vi "Init Map to Outgoing Frame Configs.vi"(7 "error in (no error)":errorcluster, 10 "RT Configuration In":T1={"Name"="", "Priority"=100, "XNET Settings"={"Database"="", "Cluster"="", "Port"="", "Baud rate [Bd]"=0, "Termination"=0, "CAN I/O Mode"=0, "FD Baud rate [Bd]"=500000, "Priority"=100, "Use Legacy"=FALSE, "FD ISO Mode"=0}, "FPGA Session"=0, "Outgoing CAN Session"="", "Outgoing Frame Count"=0, "Outgoing Frames"=[], "Incoming CAN Session"="", "Incoming Frame Count"=0, "Incoming Frames"=[], "Incoming Values"={"Signal Values"=[], "Signal Invalid Values"=[], "ProtCtr Sig Values"=[], "Timestamps"=[], "Time Differences"=[], "IDs"=[]}} {"Incoming Frames"."Protection Configurations"."CRC Channels"."Data Type" items=["Signed", "Unsigned", "IEEE Float"]; "XNET Settings"."FD ISO Mode" items=["ISO", "Non ISO", "ISO Legacy"]; "XNET Settings"."CAN I/O Mode" items=["CAN 2.0", "CAN FD", "CAN FD+BRS"]; "XNET Settings"."Termination" items=["Off", "On"]; "Outgoing Frames"."Protection Configurations"."CRC Channels"."Data Type" items=["Signed", "Unsigned", "IEEE Float"]}) -> (0 "error out":errorcluster, 2 "Map":map{i32, u8[]}(c390), 3 "RT Configuration Out":T1={"Name"="", "Priority"=100, "XNET Settings"={"Database"="", "Cluster"="", "Port"="", "Baud rate [Bd]"=0, "Termination"=0, "CAN I/O Mode"=0, "FD Baud rate [Bd]"=500000, "Priority"=100, "Use Legacy"=FALSE, "FD ISO Mode"=0}, "FPGA Session"=0, "Outgoing CAN Session"="", "Outgoing Frame Count"=0, "Outgoing Frames"=[], "Incoming CAN Session"="", "Incoming Frame Count"=0, "Incoming Frames"=[], "Incoming Values"={"Signal Values"=[], "Signal Invalid Values"=[], "ProtCtr Sig Values"=[], "Timestamps"=[], "Time Differences"=[], "IDs"=[]}} {"Incoming Frames"."Protection Configurations"."CRC Channels"."Data Type" items=["Signed", "Unsigned", "IEEE Float"]; "XNET Settings"."FD ISO Mode" items=["ISO", "Non ISO", "ISO Legacy"]; "XNET Settings"."CAN I/O Mode" items=["CAN 2.0", "CAN FD", "CAN FD+BRS"]; "XNET Settings"."Termination" items=["Off", "On"]; "Outgoing Frames"."Protection Configurations"."CRC Channels"."Data Type" items=["Signed", "Unsigned", "IEEE Float"]})   [LabVIEW 2023, in "LP_CRC.lvlib"]
uses:
  LP_CRC.lvlib
  Addon/Addon Engine/Types/RT Async Engine Settings.ctl
  Addon/Addon Shared/Types/XNET Settings.ctl
  Engine/Types/RT Frame Settings.ctl
  Shared/Types/Exported Frame Type.ctl
  Engine/Types/RT Protection Configuration.ctl
  Shared/Types/Protection Type.ctl
  Shared/Types/XNET Signal Configuration.ctl
  Shared/Types/Exported Counter Settings.ctl
  Shared/Types/Exported Event Trigger Type.ctl
  Engine/Types/RT Frame Incoming Values.ctl
  Shared/Protection and Counter Support Shared.lvlib
  Engine/Protection and Counter Support Engine.lvlib
  Addon/Addon Shared/Protection and Counter Addon Shared.lvlib
  Addon/Addon Engine/Protection and Counter Addon Engine.lvlib
panel:
  in  "key names":string[](array[string])=["22E", "2AA", "2AB", "FC", "231", "234", "E1", "22F", "232", "1A1", "13A", "CA", "DB", "316", "324", "BD", "13B", "233", "2A3", "228", "22A", "18D", "0B1", "0B2", "137", "138", "182", "183", "184", "185", "186", "18C", "227", "3CE", "FA", "FD", "25A", "B1", "B2", "B6", "B7", "2C0", "381", "181", "235", "3BA", "2AD", "2AC", "3C3", "3C2", "3C5", "305", "30B", "30C", "50", "201-214", "215-21E", "200", "21F", "52", "30", "120-12F", "14D", "190-19F", "1C0-1CF", "14C", "170-17F"]
  in  "key values":string[](array[string])=["0x8D, 0xBB, 0x4E, 0x7B, 0xE9, 0xCE, 0x31, 0x61, 0x7C, 0xB0, 0xA5, 0x3, 0x81, 0xC5, 0x84, 0x4B", "0x62, 0xB4, 0x14, 0x71, 0x7C, 0x99, 0xA1, 0xD, 0x49, 0x8B, 0x95, 0xB, 0x43, 0x94, 0x4, 0xC2", "0xD2, 0x6A, 0x4A, 0xB0, 0x9F, 0xCD, 0x65, 0x4E, 0xB4, 0xE0, 0x4C, 0x16, 0x37, 0x1C, 0xE8, 0x22", "0x8B, 0x8, 0xF1, 0x2B, 0xD3, 0x87, 0x93, 0xEE, 0x55, 0xAB, 0xC3, 0xDA, 0x91, 0x77, 0x9E, 0x3", "0x3F, 0xF1, 0xC6, 0xD5, 0xB, 0x99, 0x6F, 0xEB, 0x41, 0xF5, 0x56, 0xA2, 0xAD, 0x7, 0xCC, 0x4E", "0x45, 0xEF, 0xBA, 0xF9, 0x6B, 0xAA, 0xCC, 0x37, 0x8C, 0x74, 0x6, 0x20, 0x55, 0x5C, 0xD7, 0x57", "0x25, 0xF8, 0x32, 0xEC, 0x4F, 0x53, 0xB4, 0xC4, 0xF9, 0x30, 0x4, 0x58, 0x3E, 0x86, 0x63, 0xF6", "0x91, 0xCA, 0xEC, 0x22, 0xB2, 0xC4, 0x69, 0xCF, 0x58, 0x1B, 0x99, 0xF6, 0x9A, 0x46, 0xB9, 0xC9", "0x10, 0xBD, 0x87, 0x75, 0xF7, 0x6D, 0x42, 0x55, 0xC5, 0xC0, 0x25, 0x4C, 0xDA, 0x70, 0x40, 0x1D", "0x19, 0x8F, 0x31, 0x8D, 0x96, 0x1D, 0x67, 0x9, 0xFB, 0x66, 0xB4, 0x39, 0x10, 0xD4, 0xF6, 0xF2", "0x55, 0xAA, 0x46, 0x3C, 0x26, 0xED, 0x81, 0xCA, 0x38, 0x3E, 0xDD, 0x11, 0xA7, 0x7C, 0x1E, 0x2A", "0x98, 0x34, 0xBE, 0x86, 0x6D, 0xE, 0x89, 0x1F, 0x2B, 0x69, 0x74, 0x4D, 0xB4, 0x68, 0x44, 0x12", "0xF8, 0xBE, 0x8, 0xE, 0xF2, 0x2B, 0xC1, 0x4D, 0x87, 0x44, 0x6B, 0xEE, 0x14, 0x60, 0xAB, 0x19", "0x66, 0x7, 0x97, 0xF4, 0x23, 0x51, 0xA8, 0x2, 0x76, 0xC8, 0x8, 0x48, 0xBB, 0x52, 0x53, 0xA7", "0x2B, 0xEE, 0xDA, 0x3, 0x30, 0x32, 0x9F, 0x31, 0x3C, 0xAE, 0x5F, 0xBB, 0xD5, 0xE0, 0x33, 0x1D", "0x4C, 0xA3, 0xA1, 0x2C, 0xA4, 0x21, 0x6, 0x98, 0x97, 0x49, 0x58, 0x13, 0x28, 0x8F, 0x68, 0xDB", "0xA5, 0x5A, 0x88, 0x77, 0x50, 0x5F, 0xEF, 0xEA, 0x4D, 0x3F, 0xA3, 0xCD, 0x8E, 0xF9, 0xE1, 0x2E", "0xA5, 0xE9, 0x85, 0x4, 0xFB, 0x6C, 0xDF, 0xF1, 0xDE, 0x90, 0xA8, 0xCB, 0xDD, 0x3B, 0x80, 0x87", "0x14, 0x99, 0x49, 0xB, 0x4, 0xD5, 0x74, 0xC6, 0x17, 0xF1, 0xE1, 0x3F, 0x50, 0x9B, 0xCB, 0x10", "0xC5, 0x9E, 0x5D, 0xA1, 0xAC, 0x96, 0x1B, 0x21, 0x82, 0xEE, 0xF9, 0x97, 0xB1, 0xCB, 0xB6, 0x13", "0xD5, 0xEB, 0xA2, 0x4E, 0x35, 0xAE, 0x51, 0xCE, 0x2D, 0x79, 0x9F, 0x7C, 0x34, 0x52, 0x9, 0x3", "0x61, 0x4B, 0x17, 0xE4, 0x78, 0xB, 0xA1, 0xB4, 0xBC, 0xD8, 0xEA, 0xF5, 0xD9, 0x21, 0xCA, 0x86", "0x49, 0x56, 0xE, 0x67, 0x81, 0x1E, 0x76, 0x9F, 0xBF, 0xC1, 0xE5, 0x6C, 0x96, 0x83, 0x7F, 0xC2", "0x9C, 0xD6, 0x1C, 0xBA, 0xB8, 0x8, 0xAB, 0xAA, 0x49, 0xDF, 0x1B, 0x8C, 0x6D, 0x6E, 0xEA, 0x20", "0x57, 0x39, 0x72, 0xD, 0x51, 0xB1, 0x25, 0x28, 0x5A, 0x52, 0x85, 0xB8, 0x38, 0xF8, 0x2B, 0x6B", "0xC1, 0x5, 0xD2, 0xD9, 0xAE, 0x93, 0xB1, 0x90, 0x42, 0x7C, 0x60, 0x33, 0x46, 0xB8, 0x6A, 0xE1", "0xE8, 0x40, 0x60, 0xDE, 0xC2, 0xAC, 0xE3, 0xA4, 0x3D, 0x88, 0xD1, 0xEE, 0x51, 0x16, 0xAD, 0x49", "0xF7, 0xC0, 0x40, 0xA6, 0xA5, 0xDE, 0x62, 0x1C, 0xAC, 0x5A, 0x4F, 0xA4, 0xE5, 0x18, 0x88, 0x8", "0xD9, 0x90, 0x33, 0xE1, 0x3A, 0x1A, 0xDF, 0xC6, 0xB5, 0xDC, 0xEE, 0x4, 0xFA, 0xD7, 0xD4, 0x99", "0x5D, 0x96, 0x82, 0x97, 0xB6, 0x8B, 0x24, 0x2, 0xEB, 0x69, 0x20, 0xBB, 0x77, 0x54, 0x86, 0xE6", "0xD3, 0xE0, 0x75, 0x85, 0x83, 0x55, 0x33, 0xE3, 0x4C, 0x9C, 0x91, 0x1D, 0x23, 0x1A, 0xA6, 0x16", "0xF, 0xD1, 0x6B, 0x63, 0x9E, 0x74, 0x22, 0x94, 0xD7, 0xA1, 0xE7, 0x6F, 0x9C, 0xCF, 0x96, 0xDD", "0x66, 0xF4, 0xA8, 0xC8, 0xBB, 0xA7, 0xAF, 0x2B, 0xD9, 0x7B, 0xC0, 0x50, 0x56, 0xF, 0xCE, 0xED", "0x6C, 0x14, 0x3C, 0xAD, 0x93, 0x59, 0x1C, 0x4D, 0xD8, 0x33, 0x5D, 0x89, 0x7B, 0x8, 0x70, 0x34", "0x96, 0x97, 0x8B, 0x2, 0x69, 0xBB, 0x54, 0xE6, 0x4E, 0x46, 0x8D, 0x7B, 0xEA, 0x87, 0xE9, 0xB3", "0x53, 0x58, 0x37, 0xDA, 0x94, 0x57, 0x79, 0x27, 0x8D, 0xDD, 0xD0, 0x39, 0x16, 0x84, 0x7, 0xAF", "0x64, 0x5D, 0x7D, 0x96, 0x3D, 0x82, 0xB9, 0x97, 0xD5, 0xB6, 0xAA, 0x8B, 0x5A, 0x24, 0xB4, 0x2", "0x49, 0x56, 0xE, 0x67, 0x81, 0x1E, 0x76, 0x9F, 0xBF, 0xC1, 0xE5, 0x6C, 0x96, 0x83, 0x7F, 0xC2", "0x9C, 0xD6, 0x1C, 0xBA, 0xB8, 0x8, 0xAB, 0xAA, 0x49, 0xDF, 0x1B, 0x8C, 0x6D, 0x6E, 0xEA, 0x20", "0x71, 0xD, 0xB, 0xC2, 0x8, 0xC6, 0x63, 0x4B, 0x3F, 0x2B, 0x6, 0x10, 0xF0, 0xD2, 0x87, 0xD", "0xEB, 0x4E, 0xAE, 0xCE, 0x79, 0x7C, 0x52, 0x3, 0x6A, 0x84, 0xC2, 0x3A, 0xA, 0x64, 0x2F, 0x17", "0xA3, 0x4F, 0xD2, 0xB1, 0x60, 0x6A, 0x36, 0xF5, 0x4A, 0xAF, 0xED, 0xB0, 0x57, 0xF6, 0x9F, 0xAD", "0xB2, 0x18, 0xB8, 0xA, 0xA4, 0xD0, 0xBA, 0x5A, 0xD4, 0x54, 0x1C, 0x95, 0xB1, 0xDE, 0xD6, 0xF", "0xC8, 0x83, 0x64, 0xF, 0xC7, 0xB7, 0x3F, 0x2D, 0x68, 0x57, 0x30x, 0x88, 0x1C, 0xF7, 0x5C, 0x1A", "0xA8, 0xA7, 0xD9, 0x50, 0xCE, 0x90, 0x28, 0x3F, 0x33, 0x3, 0xDE, 0xE1, 0x1E, 0x6B, 0x3A, 0xF1", "0xB3, 0x67, 0x98, 0xD4, 0x82, 0x34, 0x53, 0x72, 0xBE, 0xF0, 0xA1, 0x86, 0x4A, 0x64, 0x6D, 0xE1", "0x31, 0x1D, 0xFB, 0x39, 0xF6, 0x90, 0x34, 0xD3, 0x80, 0x97, 0x99, 0x2F, 0x5E, 0x86, 0x1C, 0xAB", "0xE4, 0xB4, 0xF5, 0x86, 0xC, 0x35, 0x13, 0xE9, 0x5C, 0xF3, 0x5B, 0x79, 0xE1, 0x43, 0xCF, 0xB0", "0x14, 0xAD, 0x59, 0x4D, 0x33, 0x89, 0x8, 0x34, 0xC, 0x1A, 0x96, 0x11, 0x61, 0x8C, 0xB5, 0xA", "0x5, 0xD9, 0x93, 0x90, 0x7C, 0x33, 0xB8, 0xE1, 0x70, 0x3A, 0xAC, 0x1A, 0xBF, 0xDF, 0x9A, 0xC6", "0x51, 0x52, 0x2B, 0x64, 0xB3, 0xED, 0x4F, 0x5D, 0x3F, 0x80, 0xD6, 0x7D, 0xF2, 0x30, 0x4B, 0x96", "0x6A, 0xB0, 0xCD, 0x4E, 0xE0, 0x16, 0x1C, 0x22, 0x71, 0x98, 0xD9, 0xDF, 0xFA, 0x76, 0xF8, 0x14", "0x5B, 0xA8, 0x5, 0xA7, 0x4E, 0xD9, 0xD, 0x50, 0x93, 0xCE, 0x40, 0x90, 0xE, 0x28, 0x7C, 0x3F", "0xD8, 0x8E, 0x56, 0x3A, 0x18, 0xCC, 0xC9, 0x53, 0x15, 0xA, 0x90, 0x8A, 0x3E, 0x7A, 0xD0, 0x64", "0xBC, 0xEB, 0xB1, 0x41, 0x29, 0xF5, 0x66, 0x56, 0xB0, 0xA2, 0xCA, 0xAD, 0x1, 0x7, 0xB3, 0xCC", "0x27, 0xDC, 0x8D, 0x50, 0xDD, 0x9, 0xD0, 0x6D, 0x39, 0x21, 0x16, 0xF2, 0x84, 0x95, 0x7, 0x69", "0x27, 0xDC, 0x8D, 0x50, 0xDD, 0x9, 0xD0, 0x6D, 0x39, 0x21, 0x16, 0xF2, 0x84, 0x95, 0x7, 0x69", "0xF1, 0x87, 0x55, 0xDA, 0x9E, 0xAA, 0xB5, 0x32, 0x46, 0x7F, 0x2C, 0x3C, 0x7A, 0x1B, 0x26, 0xBB", "0xD9, 0xC7, 0x9A, 0x57, 0xD7, 0x5C, 0x55, 0x20, 0x6, 0x74, 0x8C, 0x37, 0xCC, 0xAA, 0x6B, 0xF9", "0x38,0x4C, 0xA, 0xD9, 0x7D, 0x5A, 0x6C, 0xC7, 0x95, 0xC4, 0x51, 0x9A, 0x41, 0xCB, 0xC0, 0x57", "0x93, 0x77, 0xB5, 0x9F, 0xB6, 0x1B, 0x41, 0xE0, 0x81, 0x27, 0x78, 0xE8, 0x6B, 0x56, 0x8F, 0x98", "0x1F, 0xB6, 0x19, 0x27, 0x9C, 0x8F, 0xA2, 0xDC, 0x31, 0xCF, 0x4A, 0x8D, 0xC2, 0xB8, 0x96, 0x50", "0xE5, 0xBA, 0xC8, 0xDE, 0xA9, 0x83, 0xB, 0xC, 0x64, 0x79, 0x44, 0xF, 0xF6, 0xC6, 0xC7, 0x5", "0x68, 0x29, 0xAF, 0xA2, 0xEF, 0xB3, 0x5B, 0xB8, 0xE0, 0x59, 0x7E, 0x67, 0x63, 0x23, 0x43, 0xD0", "0x68, 0x29, 0xAF, 0xA2, 0xEF, 0xB3, 0x5B, 0xB8, 0xE0, 0x59, 0x7E, 0x67, 0x63, 0x23, 0x43, 0xD0", "0x6C, 0xCB, 0xC, 0x55, 0xEA, 0x5, 0x4B, 0xAA, 0x2D, 0x28, 0x9C, 0x46, 0xF4, 0x84, 0x1, 0x3C", "0x1F, 0xB6, 0x19, 0x27, 0x9C, 0x8F, 0xA2, 0xDC, 0x31, 0xCF, 0x4A, 0x8D, 0xC2, 0xB8, 0x96, 0x50"]
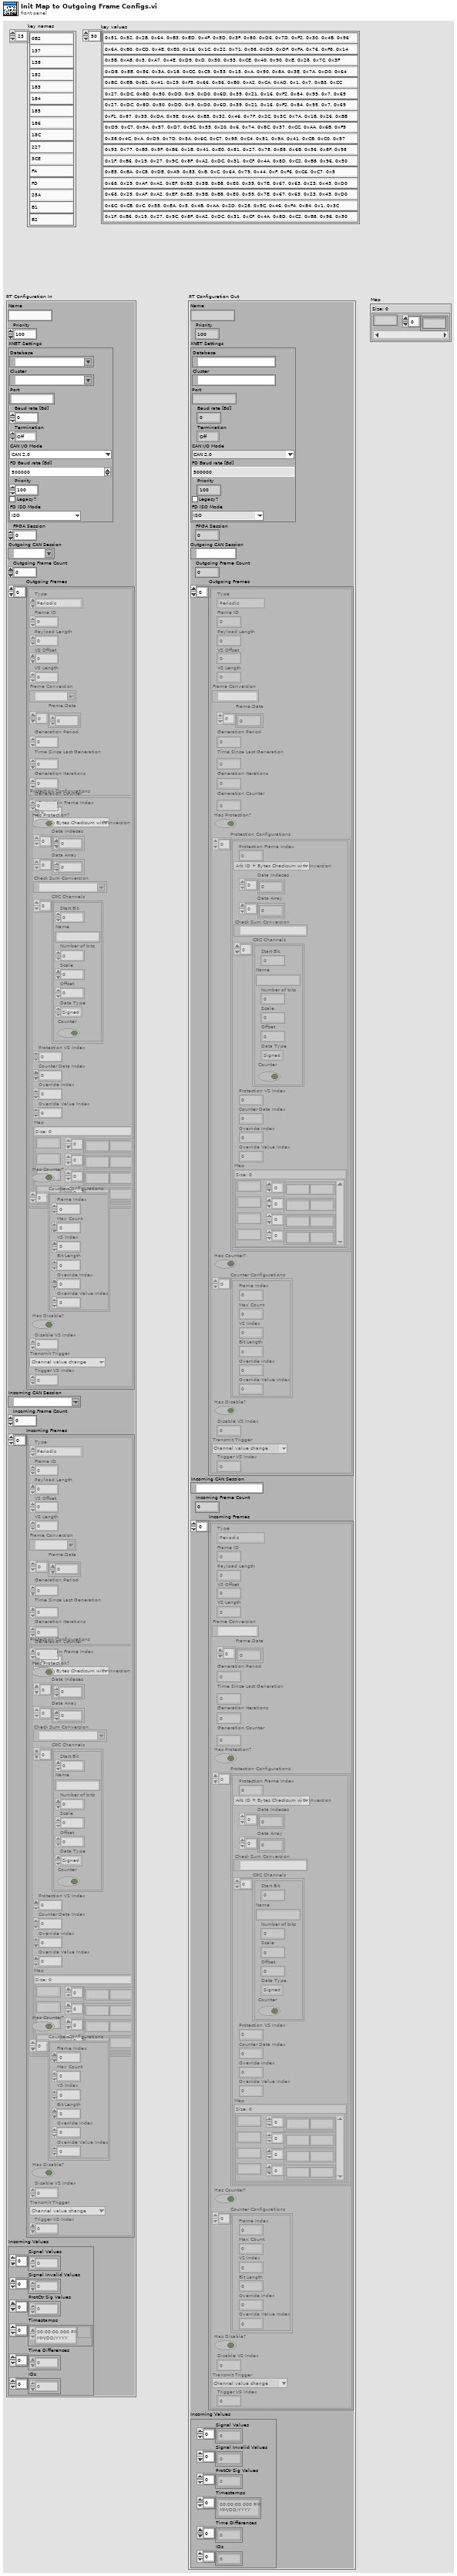
[diagram p1: front panel]
types:
  T1 = typedef "Protection and Counter Addon Engine.lvlib/RT Async Engine Settings.ctl" = cluster{"Name":string, "Priority":i32, "XNET Settings":T2, "FPGA Session":u32, "Outgoing CAN Session":refnum<k21>, "Outgoing Frame Count":i32, "Outgoing Frames":T3[], "Incoming CAN Session":refnum<k21>, "Incoming Frame Count":i32, "Incoming Frames":T3[], "Incoming Values":T10}
  T2 = typedef "Protection and Counter Addon Shared.lvlib/XNET Settings.ctl" = cluster{"Database":refnum<k21>, "Cluster":refnum<k21>, "Port":string, "Baud rate [Bd]":u64, "Termination":u32, "CAN I/O Mode":u32, "FD Baud rate [Bd]":u64, "Priority":i32, "Use Legacy":bool, "FD ISO Mode":u32}
  T3 = typedef "Protection and Counter Support Engine.lvlib/RT Frame Settings.ctl" = cluster{"Type":T4, "Frame ID":u32, "Payload Length":u32, "VS Offset":i32, "VS Length":i32, "Frame Conversion":refnum<k21>, "Frame.Data":dbl[], "Generation Period":u32, "Time Since Last Generation":u32, "Generation Iterations":u32, "Generation Counter":u32, "Has Protection?":bool, "Protection Configurations":T5[], "Has Counter?":bool, "Counter Configurations":T8[], "Has Disable?":bool, "Disable VS Index":i32, "Transmit Trigger":T9, "Trigger VS Index":i32}
  T4 = typedef "Protection and Counter Support Shared.lvlib/Exported Frame Type.ctl" = enum16{"Periodic", "Event", "Periodic/Event"}
  T5 = typedef "Protection and Counter Support Engine.lvlib/RT Protection Configuration.ctl" = cluster{"Protection Frame Index":i32, "Protection Type":T6, "Data Indeces":i32[], "Data Array":dbl[], "Check Sum Conversion":refnum<k21>, "CRC Channels":T7[], "Protection VS Index":i32, "Counter Data Index":i32, "Override Index":i32, "Override Value Index":i32, "Map":map{i32, u8[]}}
  T6 = typedef "Protection and Counter Support Shared.lvlib/Protection Type.ctl" = enum16{"Arb ID + Bytes Checksum with Inversion", "Arb ID + Bytes CRC with Inversion", "Reversed Raw Signal Checksum with Inversion", "Concatenated Two's Compliment", "LP_CRC8", "LP_Checksum", "LP_CRC8_MRS"}
  T7 = typedef "Protection and Counter Support Shared.lvlib/XNET Signal Configuration.ctl" = cluster{"Start Bit":i32, "Name":string, "Number of bits":i32, "Scale":dbl, "Offset":dbl, "Data Type":u32, "Counter":bool}
  T8 = typedef "Protection and Counter Support Shared.lvlib/Exported Counter Settings.ctl" = cluster{"Frame Index":i32, "Max Count":dbl, "VS Index":i32, "Bit Length":i64, "Override Index":i32, "Override Value Index":i32}
  T9 = typedef "Protection and Counter Support Shared.lvlib/Exported Event Trigger Type.ctl" = enum16{"Channel value change", "Trigger channel (not zero)", "Channel value change or trigger channel (not zero)", "Trigger channel (any value change)", "Channel value change or trigger channel (any value change)"}
  T10 = typedef "Protection and Counter Support Engine.lvlib/RT Frame Incoming Values.ctl" = cluster{"Signal Values":dbl[], "Signal Invalid Values":dbl[], "ProtCtr Sig Values":dbl[], "Timestamps":timestamp[], "Time Differences":dbl[], "IDs":u32[]}
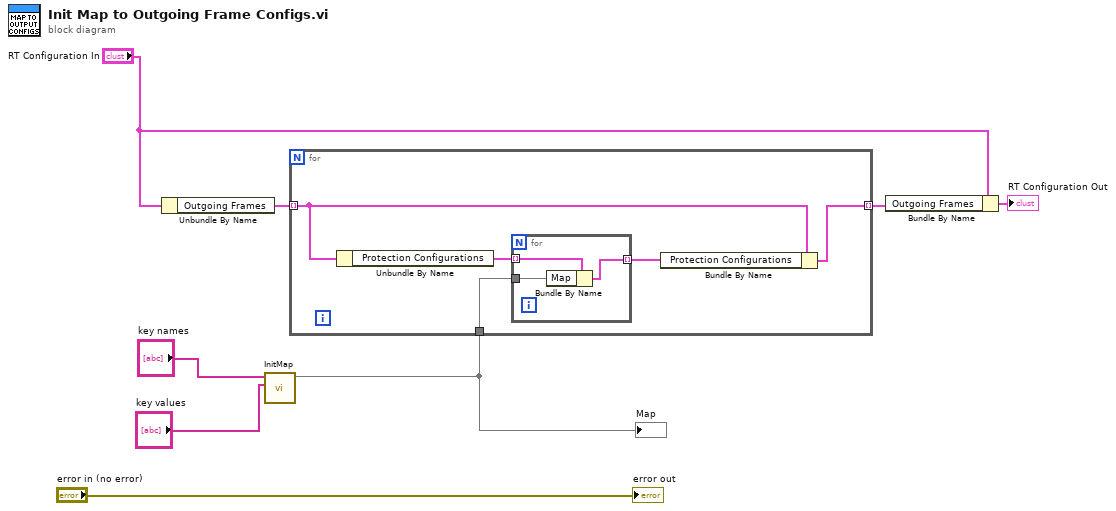
[diagram p0: block diagram]
diagram:
  n1 = Unbundle By Name("RT Configuration In") -> ("Outgoing Frames"=w5:T3[])
  n2 = call "InitMap.vi"("key values"="key values", "key names"="key names") -> ("Map"=w2:map{i32, u8[]})  [unwired: 9 in]
  "Map" <- w2
  n3 = for {
    tunnel: w5 -> [w12] mode=indexing
    tunnel: [w10] -> w3 mode=indexing
    tunnel: w2 -> [w9]
    n4 = Unbundle By Name(w12) -> ("Protection Configurations"=w13:T5[])
    n5 = for {
      tunnel: w13 -> [w16] mode=indexing
      tunnel: [w15] -> w11 mode=indexing
      tunnel: w9 -> [w14]
      n6 = Bundle By Name(cluster=w16, "Map"=w14) -> (w15:T5)
    }
    n7 = Bundle By Name(cluster=w12, "Protection Configurations"=w11) -> (w10:T3)
  }
  n8 = Bundle By Name(cluster="RT Configuration In", "Outgoing Frames"=w3) -> (→"RT Configuration Out":T1)
  "error out" <- "error in (no error)"
